vi "hcVVV.vi"() -> ()   [LabVIEW 2014]
panel:
  out "I":i32
  out "Id":dbl
  out "II":dbl
  out "m":i32
  out "p":i32
  out "n":i32
  out "oneD":bool
  out "Error Message":string
  out "hcPair":dbl[][](array[numeric])
  in  "beta":dbl=1.0
  in  "alpha":dbl=1.0
  in  "minclus":i32=1
  in  "partition":i32[](array[numeric])
  in  "data":dbl[][](array[numeric])
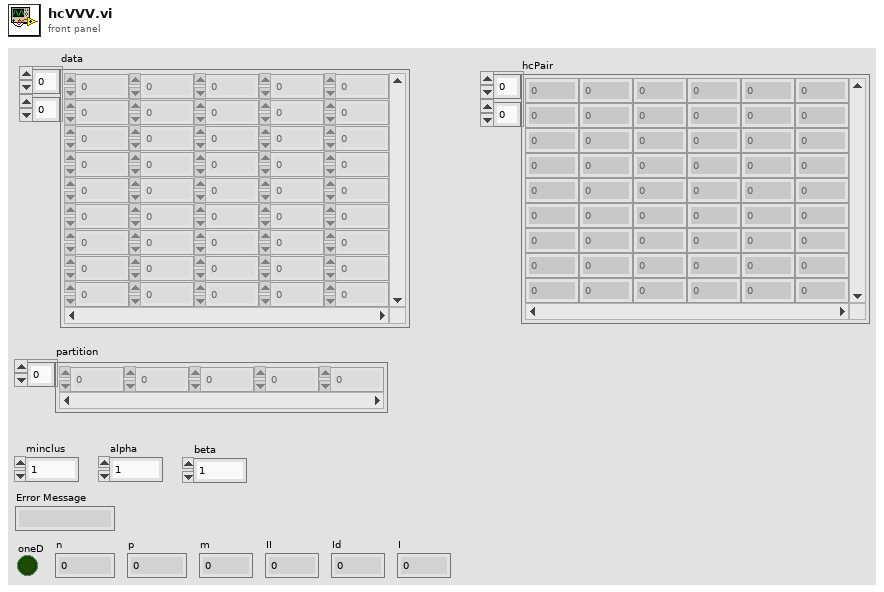
[diagram p1: front panel]
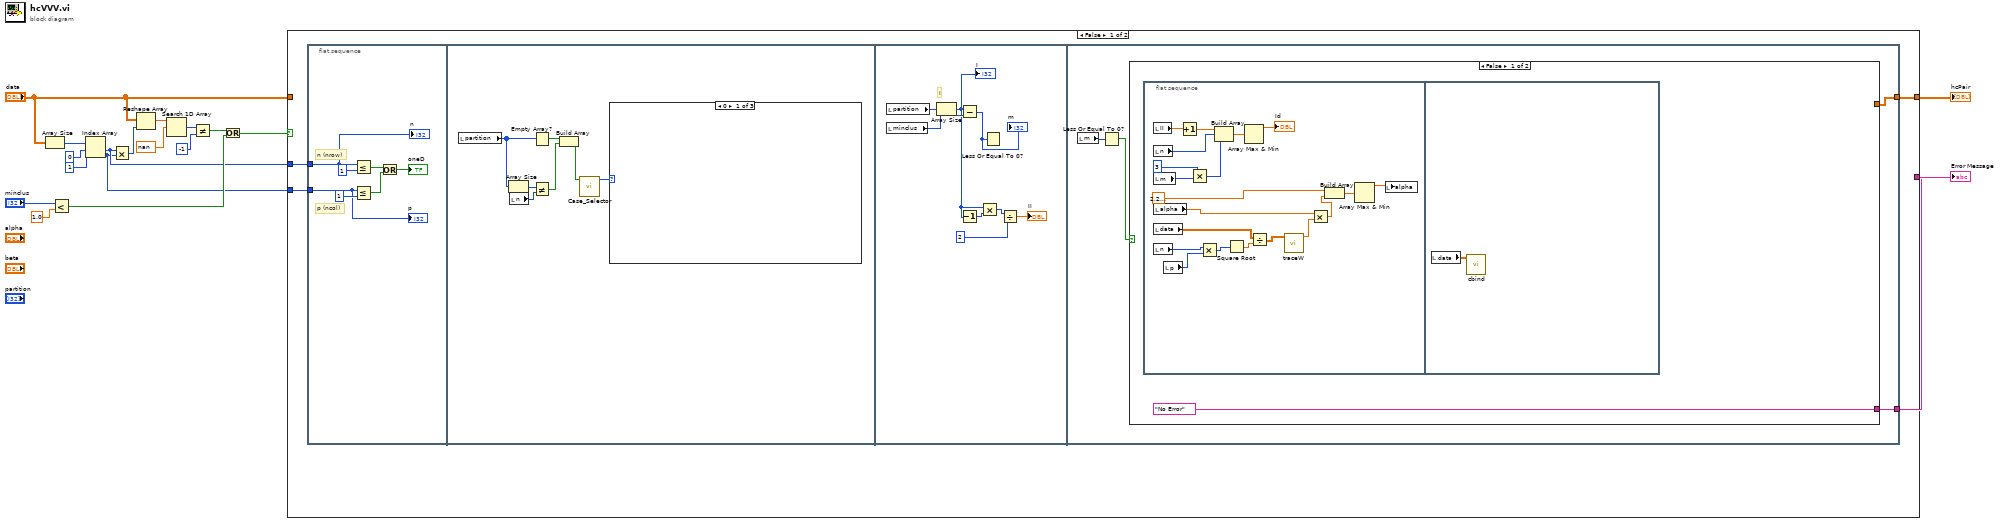
[diagram p0: block diagram]
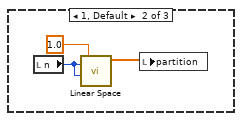
[diagram p2: hidden frame]
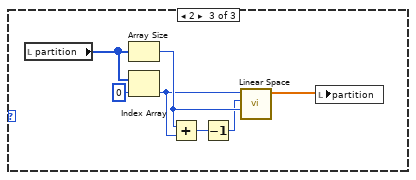
[diagram p3: hidden frame]
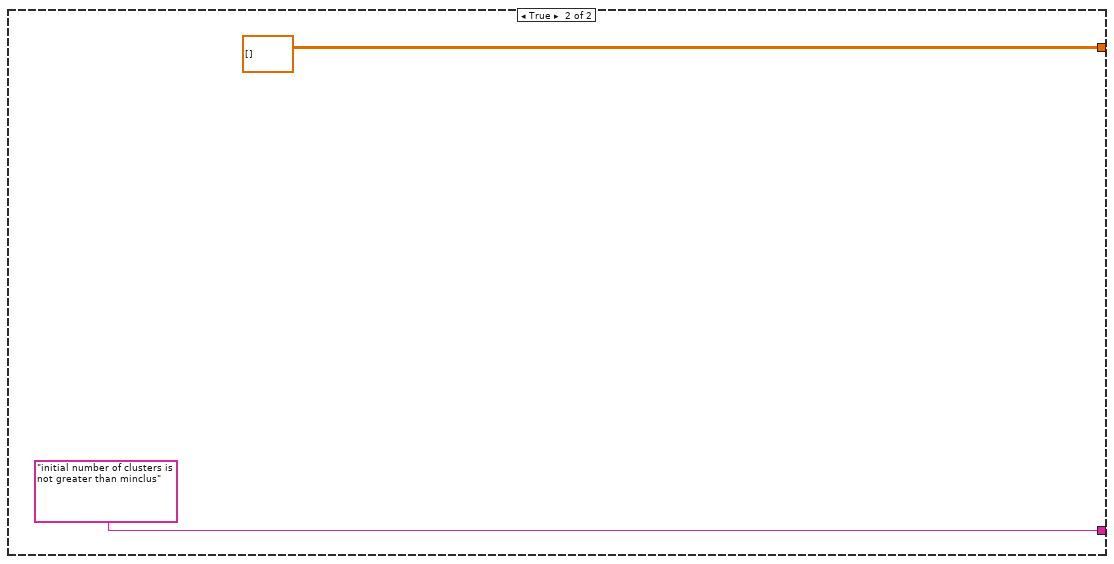
[diagram p4: hidden frame]
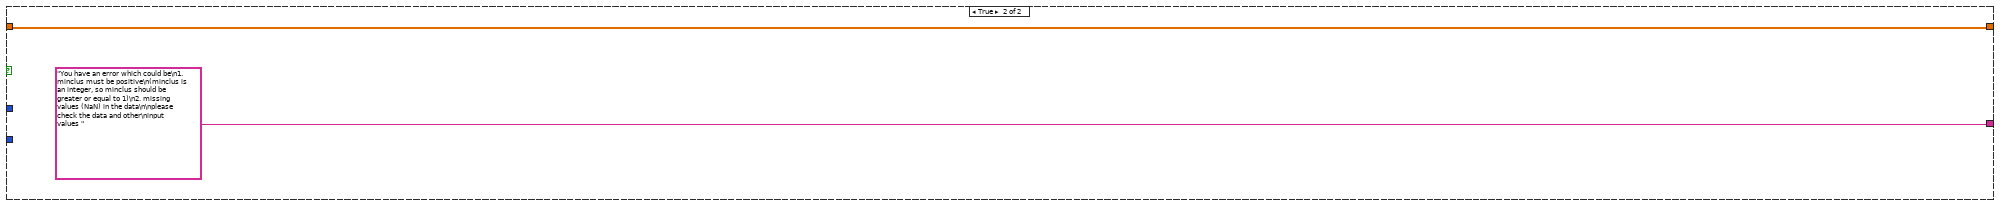
[diagram p5: hidden frame]
diagram:
  n1 = Array Size(array="data") -> (size(s)=w5:i32[])
  n2 = Less?(x="minclus", y=1.0) -> (x < y?=w10:bool)
  n3 = Index Array(array=w5, index #1=0 ("index"), index #2=1 ("index")) -> (element #1=w3:i32, element #2=w1:i32)
  n4 = Multiply(x=w3, y=w1) -> (x*y=w16:i32)
  n5 = Reshape Array("data", w16) -> (w15:dbl[])
  n6 = Search 1D Array(1D array=w15, element=nan) -> (index of element=w13:i32)  [unwired: 1 in]
  n7 = Not Equal?(x=w13, y=-1) -> (x != y?=w11:bool)
  n8 = Or(x=w11, y=w10) -> (x .or. y?=w9:bool)
  n9 = case shown="False" w9 {
    tunnel: "data" -> [_ w84]
    tunnel: [w20 w84] -> w7
    tunnel: [w19 "You have an error which could be\n1. minclus must be positive\n(minclus is an integer, so minclus should be greater or equal to 1)\n2. missing values (NaN) in the data\n\nplease check the data and other\ninput values "] -> w6
    tunnel: w3 -> [w22 _]
    tunnel: w1 -> [w21 _]
    frame False {
      n10 = flat-sequence {
        tunnel: w22 -> [w29]
        tunnel: w21 -> [w23]
        tunnel: [w56] -> w20
        tunnel: [w55] -> w19
        frame #0 {
          # "p (ncol)"
          # "n (nrow)"
          n11 = Less Or Equal?(x=w29, y=1) -> (x <= y?=w26:bool)
          n12 = Less Or Equal?(x=w23, y=1) -> (x <= y?=w25:bool)
          n13 = Or(x=w26, y=w25) -> (x .or. y?=→"oneD":bool)
          "n" <- w29
          "p" <- w23
        }
        frame #1 {
          n14 = local read "partition"() -> (w36:i32[])
          n15 = Array Size(array=w36) -> (size(s)=w34:i32)
          n16 = local read "n"() -> (w35:i32)
          n17 = Empty Array?(array=w36) -> (empty?=w33:bool)
          n18 = Not Equal?(x=w34, y=w35) -> (x != y?=w32:bool)
          n19 = Build Array(w33, w32) -> (w31:bool[])
          n20 = call "Case_Selector.vi"("Array"=w31) -> ("Case Numer"=w30:i32)  [unwired: 10 in]
          n21 = case shown="0" w30 {
            frame 0 {
            }
            frame 1, Default {
              n22 = local read "n"() -> (w37:i32)
              n23 = call "Linear Space.vi"("Number of Samples"=w37, "Maximum"=w37, "Minimum"=1.0) -> ("Array"=w39:dbl[])  [unwired: 3 in, 1 out]
              n24 = local write "partition"(w39) -> ()
            }
            frame 2 {
              n25 = local read "partition"() -> (w40:i32[])
              n26 = Array Size(array=w40) -> (size(s)=w45:i32)
              n27 = Index Array(array=w40, index=0) -> (element=w44:i32)
              n28 = Add(x=w45, y=w44) -> (x+y=w43:i32)
              n29 = Decrement(x=w43) -> (x-1=w42:i32)
              n30 = call "Linear Space.vi"("Number of Samples"=w45, "Maximum"=w42, "Minimum"=w44) -> ("Array"=w41:dbl[])  [unwired: 3 in, 1 out]
              n31 = local write "partition"(w41) -> ()
            }
          }
        }
        frame #2 {
          # "I"
          n32 = local read "partition"() -> (w54:i32[])
          n33 = local read "minclus"() -> (w53:i32)
          n34 = Array Size(array=w54) -> (size(s)=w50:i32)
          "I" <- w50
          n35 = Subtract(x=w50, y=w53) -> (x-y=w52:i32)
          "m" <- w52
          n36 = Decrement(x=w50) -> (x-1=w51:i32)
          n37 = Multiply(x=w50, y=w51) -> (x*y=w49:i32)
          n38 = Less Or Equal To 0?(x=w52) -> ()  [unwired: 1 out]
          n39 = Divide(x=w49, y=2) -> (x/y=→"II":dbl)
        }
        frame #3 {
          n40 = local read "m"() -> (w58:i32)
          n41 = Less Or Equal To 0?(x=w58) -> (x <= 0?=w57:bool)
          n42 = case shown="False" w57 {
            tunnel: [_ dbl[][] [] ("data")] -> w56
            tunnel: ["No Error" "initial number of clusters is not greater than minclus"] -> w55
            frame False {
              n43 = flat-sequence {
                frame #0 {
                  n44 = local read "II"() -> (w77:dbl)
                  n45 = local read "n"() -> (w79:i32)
                  n46 = local read "m"() -> (w76:i32)
                  n47 = local read "alpha"() -> (w71:dbl)
                  n48 = local read "data"() -> (w66:dbl[][])
                  n49 = local read "n"() -> (w69:i32)
                  n50 = local read "p"() -> (w70:i32)
                  n51 = Increment(x=w77) -> (x+1=w78:dbl)
                  n52 = Multiply(x=3, y=w76) -> (x*y=w74:i32)
                  n53 = Multiply(x=w69, y=w70) -> (x*y=w68:i32)
                  n54 = Build Array(w78, w79, w74) -> (w73:dbl[])
                  n55 = Square Root(x=w68) -> (sqrt(x)=w67:dbl)
                  n56 = Array Max & Min(array=w73) -> (max value=→"Id":dbl)  [unwired: 3 out]
                  n57 = Divide(x=w66, y=w67) -> (x/y=w65:dbl[][])
                  n58 = call "traceW.vi"("x"=w65) -> ("ss"=w64:dbl)  [unwired: 10 in]
                  n59 = Multiply(x=w71, y=w64) -> (x*y=w63:dbl)
                  n60 = Build Array(2.220446049250313e-16, w63) -> (w61:dbl[])
                  n61 = Array Max & Min(array=w61) -> (max value=w60:dbl)  [unwired: 3 out]
                  n62 = local write "alpha"(w60) -> ()
                }
                frame #1 {
                  n63 = local read "data"() -> (w80:dbl[][])
                  n64 = call "cbind.vi"("data"=w80) -> ()  [unwired: 10 in, 1 out]
                }
              }
            }
            frame True {
            }
          }
        }
      }
    }
    frame True {
    }
  }
  "hcPair" <- w7
  "Error Message" <- w6
